vi "read_basic_log.vi"(11 "refnum out":refnum<file>) -> (2 "Array of gathered data in a cluster":T1[](array[typedef]) {"SailPositions"."MainSailSuggestion" min=0.0 max=1.0; "SailPositions"."JibSailSuggestion" min=0.0 max=1.0; "RudderPosition" min=-0.95 max=0.95 scale=1.0..-1.0; "BoatLocation"."North" format="%#_10f"; "BoatLocation"."East" format="%#_8f"}, 3 "size(s)":i32)   [LabVIEW 2013]
doc: "Reads the message created by write_basic_log IF the saved variables and the \"read\" variables are the same.\n\nEric Schneider, October 2014"
uses:
  Data/TypeDefs/BasicLogReading.ctl
  Data/TypeDefs/Sail Set Suggestions.ctl
  Data/TypeDefs/Rudder Set Suggestions.ctl
  Data/TypeDefs/UTM Location.ctl
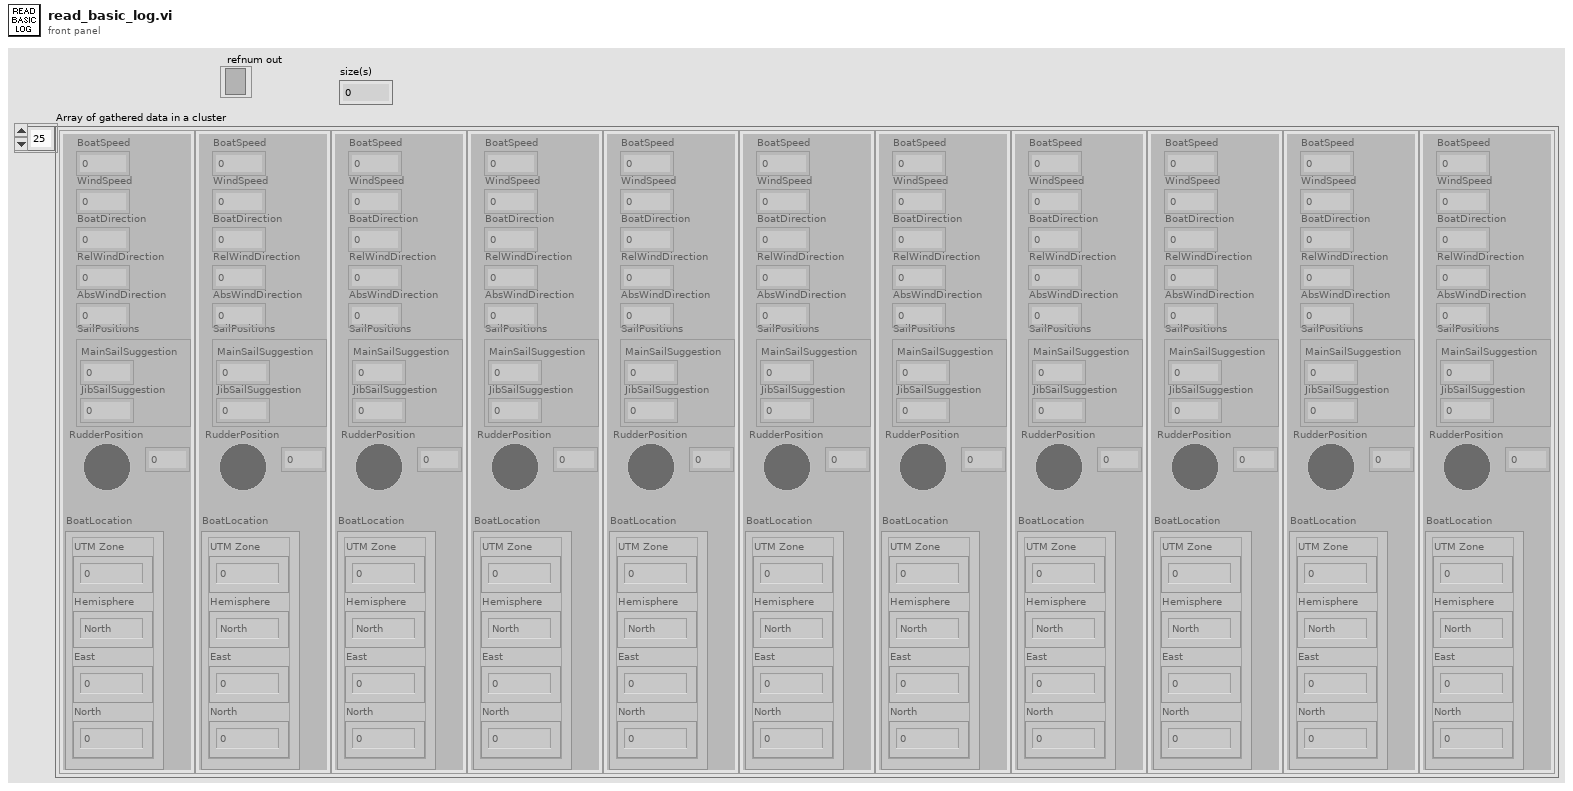
[diagram p1: front panel]
types:
  T1 = typedef "BasicLogReading.ctl" = cluster{"BoatSpeed":dbl, "WindSpeed":dbl, "BoatDirection":dbl, "RelWindDirection":dbl, "AbsWindDirection":dbl, "SailPositions":T2, "RudderPosition":T3, "BoatLocation":T4}
  T2 = typedef "Sail Set Suggestions.ctl" = cluster{"MainSailSuggestion":dbl, "JibSailSuggestion":dbl}
  T3 = typedef "Rudder Set Suggestions.ctl" = dbl
  T4 = typedef "UTM Location.ctl" = cluster{"UTM Zone":dbl, "Hemisphere":enum16{"North", "South"}, "East":dbl, "North":dbl}
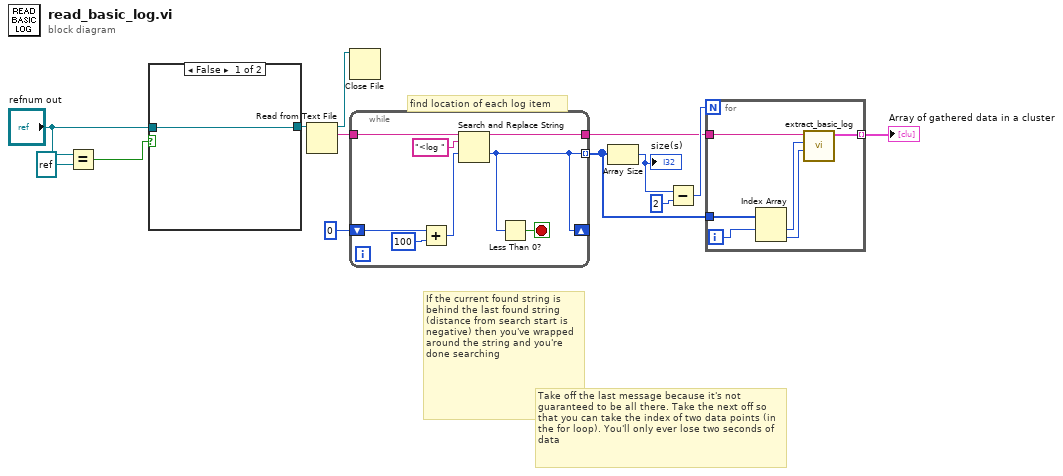
[diagram p0: block diagram]
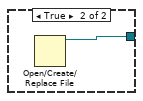
[diagram p2: hidden frame]
diagram:
  # "Take off the last message because it's not guaranteed to be all there. Take the next off so that you can take the index of two data points (in the for loop). You'll only ever lose two seconds of data"
  # "If the current found string is behind the last found string (distance from search start is negative) then you've wrapped around the string and you're done searching"
  # "find location of each log item"
  n1 = Equal?(x="refnum out", y=refnum<file> refnum) -> (x = y?=w2:bool)
  n2 = case shown="False" w2 {
    tunnel: [w14 w15] -> w13
    tunnel: "refnum out" -> [w14 _]
    frame False {
    }
    frame True {
      n3 = Open/Create/Replace File() -> (refnum out=w15:refnum<file>)  [unwired: 6 in, 2 out]
    }
  }
  n4 = Read from Text File(file (use dialog)=w13) -> (refnum out=w12:refnum<file>, text=w11:string)  [unwired: 3 in, 2 out]
  n5 = Close File(refnum=w12) -> ()  [unwired: 1 in, 2 out]
  n6 = while {
    tunnel: w11 -> [w23]
    shift-right: [w16] -> _
    shift-left: 0 ("offset past replacement") -> [w20]
    tunnel: [w17] -> w5
    tunnel: [w16] -> w6 mode=indexing
    stop <- w21 stop-if-true
    n7 = Add(x=w20, y=100) -> (x+y=w19:i32)
    n8 = Search and Replace String(input string=w23, search string="<log ", offset=w19) -> (result string=w17:string, offset past replacement=w16:i32)  [unwired: 5 in, 2 out]
    n9 = Less Than 0?(x=w16) -> (x < 0?=w21:bool)
  }
  n10 = Array Size(array=w6) -> (size(s)=w9:i32)
  "size(s)" <- w9
  n11 = Subtract(x=w9, y=2) -> (x-y=w7:i32)
  n12 = for {
    N: w7 -> [_]
    tunnel: w6 -> [w29]
    tunnel: w5 -> [w28]
    tunnel: [w25] -> w4 mode=indexing
    i -> [w24]
    n13 = Index Array(array=w29, index #1=w24) -> (element #1=w27:i32, element #2=w26:i32)  [unwired: 1 in]
    n14 = call "extract_basic_log.vi"("Next element index"=w26, "Current element index"=w27, "total string"=w28) -> ("Cluster of named data"=w25:T1)  [unwired: 8 in]
  }
  "Array of gathered data in a cluster" <- w4
